vi "ARMA Prediction.vi"() -> ()   [LabVIEW 2023]
doc: "This example shows how to obtain AR model parameters of a univariate time series using the TSA AR Model Estimation VI, then use the TSA ARMA Prediction VI to forecasts the future values of the time series.\n\n<b>Instructions:</b>\n1) Run this VI.\n2) Compare the predicted record and the real record."
uses:
  <vilib>/addons/Time Series Analysis/Modeling and Prediction.llb/TSA AR Modeling (Array).vi
  <vilib>/addons/Time Series Analysis/Statistical Analysis.llb/TSA Deviation and Variance (Array).vi
  <vilib>/addons/Time Series Analysis/Modeling and Prediction.llb/TSA ARMA Prediction (Array).vi
  <vilib>/addons/_Advanced Signal Processing/NI_AdvSigProcTSA.lvlib
  <vilib>/Analysis/NI_AALPro.lvlib
panel:
  out "Confidence level (%)":dbl format="%.2f"
  in  "Number of predictions":i32=12
  in  "AR order":i32=60
  out "Prediction Result":dbl[][](graph)
  out "Original Temperature":dbl[](graph)
  in  "stop":bool
  # "Overview: Shows how to obtain AR model parameters of a univariate time series using the TSA AR ModelingVI, then use the TSA ARMA Prediction VI to forecasts the future values of the time series.\nRequirements: LabVIEW Full Development System, Advanced Signal Processing Toolkit\nInstructions: \n1. Run this VI.\n2. Compare the predicted record and the real record.\n3. Click Stop to stop the VI."
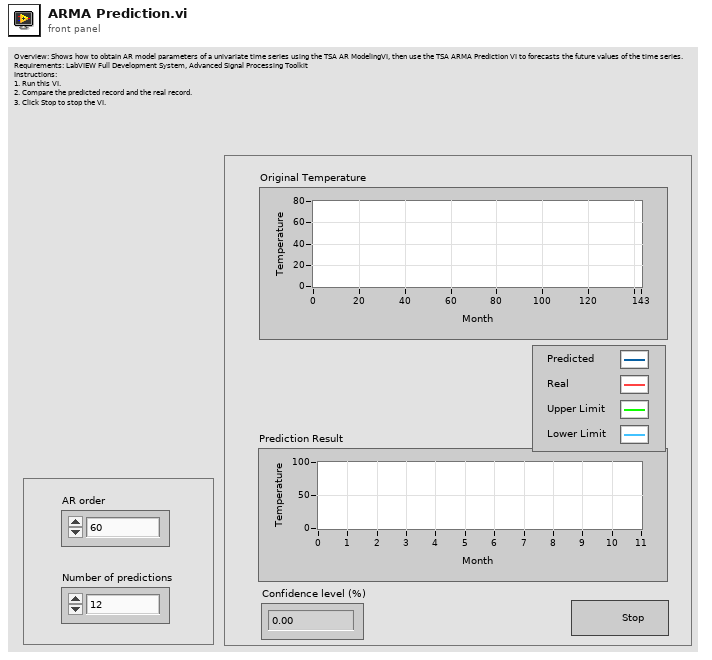
[diagram p1: front panel]
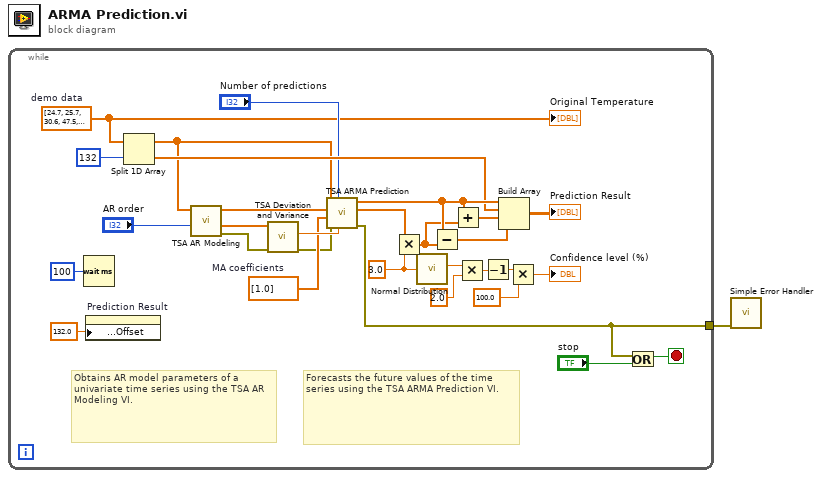
[diagram p0: block diagram]
diagram:
  n1 = while {
    tunnel: [w2] -> w1
    stop <- w30 stop-if-true
    w12 = 3.0
    w15 = dbl[] [24.7, 25.7, 30.6, 47.5, 62.9, 68.5, 73.7, 67.9, 61.1, 48.5, 39.6, 20.0, 16.1, 19.1, 24.2, 45.4, 61.3, 66.5, 72.1, 68.4, 60.2, 50.9, 37.4, 31.1, 10.4, 21.6, 37.4, 44.7, 53.2, 68.0, 73.7, 68.2, 60.7, 50.2, 37.2, 24.6, 21.5, 14.7, 35.0, 48.3, 54.0, 68.2, 69.6, 65.7, 60.8, 49.1, 33.2, 26.0, 19.1, 20.6, 40.2, 50.0, 55.3, 67.7, 70.7, 70.3, 60.6, 50.7, 35.8, 20.7, 14.0, 24.1, 29.4, 46.6, 58.6, 62.2, 72.1, 71.7, 61.9, 47.6, 34.2, 20.4, 8.4, 19.0, 31.4, 48.7, 61.6, 68.1, 72.2, 70.6, 62.5, 52.7, 36.7, 23.8, 11.2, 20.0, 29.6, 47.7, 55.8, 73.2, 68.0, 67.1, 64.9, 57.1, 37.6, 27.7, 13.4, 17.2, 30.8, 43.7, 62.3, 66.4, 70.2, 71.6, 62.1, 46.0, 32.7, 17.3, 22.5, 25.7, 42.3, 45.2, 55.5, 68.9, 72.3, 72.3, 62.5, 55.6, 38.0, 20.4, 17.6, 20.5, 34.2, 49.2, 54.8, 63.8, 74.0, 67.1, 57.7, 50.8, 36.8, 25.5, 20.4, 19.6, 24.6, 41.3, 61.8, 68.5, 72.0, 71.1, 57.3, 52.5, 40.6, 26.2]  # demo data
    w17 = dbl[] [1.0]  # MA coefficients
    # "Forecasts the future values of the time series using the TSA ARMA Prediction VI."
    # "Obtains AR model parameters of a univariate time series using the TSA AR Modeling VI."
    n2 = Wait (ms)(milliseconds to wait=u32 100 ("millisecond multiple")) -> ()  [unwired: 1 out]
    n3 = property on="Prediction Result" class="WFGraph (strict)"("X Scale.Offset and Multiplier:Offset"=132.0) -> ()  [unwired: 2 in, 2 out]
    n4 = Split 1D Array(array=w15, index=132) -> (first subarray=w13:dbl[], second subarray=w20:dbl[])
    n5 = call-poly <vilib>:"TSA AR Modeling.vi"("AR order"="AR order", "Xt"=w13) -> ("error out"=w4:errorcluster, "noise"=w24:dbl[], "AR coefficients"=w28:dbl[])  [unwired: 2 in, 5 out]
    n6 = call-poly <vilib>:"TSA Deviation and Variance.vi"("error in (no error)"=w4, "Xt"=w24) -> ("error out"=w3:errorcluster, "variance"=w25:dbl)  [unwired: 1 in, 7 out]
    n7 = call-poly <vilib>:"TSA ARMA Prediction.vi"("noise variance"=w25, "number of points"="Number of predictions", "error in (no error)"=w3, "MA coefficients"=w17, "AR coefficients"=w28, "Xt"=w13) -> ("error out"=w2:errorcluster, "standard deviation"=w18:dbl[], "predicted series"=w23:dbl[])  [unwired: 3 out]
    n8 = Multiply(x=w18, y=w12) -> (x*y=w19:dbl[])
    n9 = call <vilib>:"Normal Distribution.vi"("x"=w12) -> ("probability"=w11:dbl)
    n10 = Subtract(x=w23, y=w19) -> (x-y=w14:dbl[])
    n11 = Add(x=w23, y=w19) -> (x+y=w26:dbl[])
    n12 = Multiply(x=w11, y=2.0) -> (x*y=w10:dbl)
    n13 = Decrement(x=w10) -> (x-1=w8:dbl)
    n14 = Build Array(w23, w20, w26, w14) -> (→"Prediction Result":dbl[][])
    n15 = Multiply(x=w8, y=100.0) -> (x*y=→"Confidence level (%)":dbl)
    n16 = Or(x=w2, y="stop") -> (x .or. y?=w30:bool)
    "Original Temperature" <- w15
  }
  n17 = call <vilib>:"Simple Error Handler.vi"("error in (no error)"=w1) -> ()  [unwired: 1 in, 8 out]
